vi "Finish.vi"   [LabVIEW 2011]
doc: "This VI is called just before exiting. It is expected to close I/O refnum, save collected data, etc."
types:
  T1 = typedef "WPI_JoystickDevRef.ctl" = cluster{"Device":T2}
  T2 = typedef "WPI_JoystickDeviceEnum.ctl" = enum16{"USB 1", "USB 2", "USB 3", "USB 4", "Kinect 1", "Kinect 2"}
  T3 = typedef "WPI_MotorControlDeviceRef.ctl" = cluster{"DeviceStatus":errorcluster, "Type":enum16{"PWM", "CAN"}, "PWM":cluster{"Digital Module":T4, "PWM Channel":T5, "DeadBand":T6}, "CAN":cluster{"Device Number":u8, "Control Mode":T7, "Semaphore":T8, "Max Vout":dbl}, "Invert":bool, "TransformRef":T9, "InvTransformRef":T9}
  T4 = typedef "FPGA_TypedefDigitalModule.ctl" = enum16{"Digital Module 1", "Digital Module 2"}
  T5 = typedef "FPGA_DIOPWMChannel.ctl" = enum8{"PWM 1", "PWM 2", "PWM 3", "PWM 4", "PWM 5", "PWM 6", "PWM 7", "PWM 8", "PWM 9", "PWM 10", "Invalid"}
  T6 = typedef "WPI_PWMDeadband.ctl" = cluster{"Name":string, "maxPositivePwm":i32, "minPositivePwm":i32, "centerPwm":i32, "maxNegativePwm":i32, "minNegativePwm":i32, "angularRange":u16}
  T7 = typedef "WPI_CANJaguar_ControlMode.ctl" = enum8{"Percent VBus", "Current", "Speed", "Position", "Voltage"}
  T8 = typedef "Semaphore RefNum" = refnum<k1>
  T9 = typedef "WPI_PWMTransform_ConPane.ctl" = refnum<vi>
  T10 = typedef "WPI_AnalogChannelDevRef.ctl" = cluster{"DevStatus":errorcluster, "Analog Module":T11, "Analog Channel":T12}
  T11 = typedef "FPGA_TypedefAnalogModule.ctl" = enum16{"Analog Module 1", "Analog Module 2"}
  T12 = typedef "FPGA_AIChannel.ctl" = enum8{"AI 1", "AI 2", "AI 3", "AI 4", "AI 5", "AI 6", "AI 7", "AI 8", "Invalid"}
  T13 = typedef "WPI_RelayDevRef.ctl" = cluster{"DevStatus":errorcluster, "Relay Channel":T14, "Digital Module":T4, "Relay Direction":T15}
  T14 = typedef "FPGA_DIORelayChannel.ctl" = enum8{"Relay 1", "Relay 2", "Relay 3", "Relay 4", "Relay 5", "Relay 6", "Relay 7", "Relay 8", "Invalid"}
  T15 = typedef "WPI_RelayDirection.ctl" = enum16{"Both directions", "Forward only", "Reverse only"}
  T16 = typedef "WPI_RobotDriveDevRef.ctl" = cluster{"DevStatus":errorcluster, "Motors[]":T3[], "Square Inputs":bool, "Max Output":dbl, "Isochronous":bool}
  T17 = typedef "WPI_CameraDevRef.ctl" = cluster{"Camera Address":string, "CameraStatus":errorcluster, "Acquire Image Notifier":refnum<notifier>}
  T18 = typedef "WPI_ServoDeviceRef.ctl" = cluster{"DeviceStatus":errorcluster, "Digital Module":T4, "PWM Channel":T5, "DeadBand":T6}
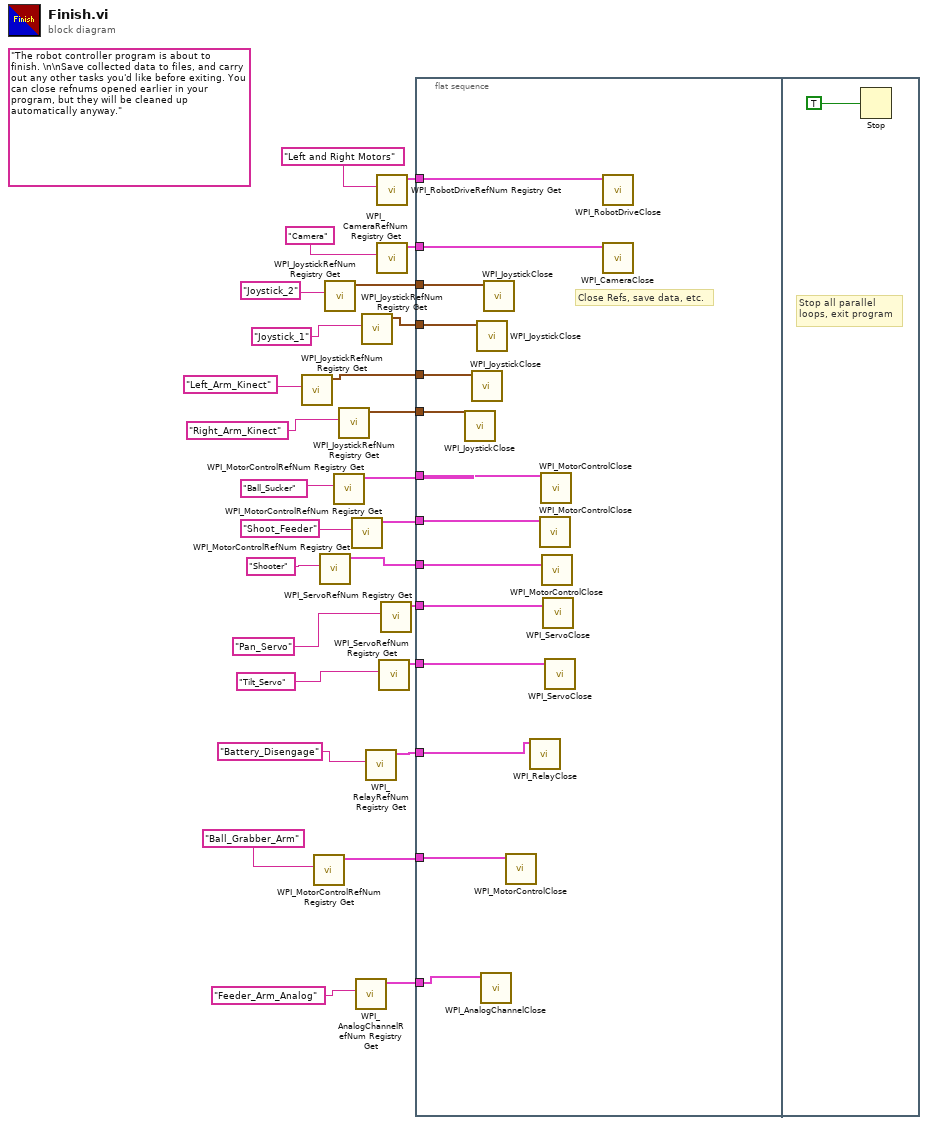
[diagram p0: block diagram]
diagram:
  (unwired) "The robot controller program is about to finish. \n\nSave collected data to files, and carry out any other tasks you'd like before exiting. You can close refnums opened earlier in your program, but they will be cleaned up automatically anyway."
  n1 = call <vilib>:"WPI_JoystickRefNum Registry Get.vi"("refnum name"="Left_Arm_Kinect") -> ("JoystickDevRef"=w6:T1)  [unwired: 1 in, 9 out]
  n2 = call <vilib>:"WPI_MotorControlRefNum Registry Get.vi"("refnum name"="Ball_Grabber_Arm") -> ("MotorControlDevRef"=w3:T3)  [unwired: 9 in, 1 out]
  n3 = call <vilib>:"WPI_MotorControlRefNum Registry Get.vi"("refnum name"="Shooter") -> ("MotorControlDevRef"=w17:T3)  [unwired: 9 in, 1 out]
  n4 = call <vilib>:"WPI_JoystickRefNum Registry Get.vi"("refnum name"="Joystick_2") -> ("JoystickDevRef"=w23:T1)  [unwired: 1 in, 9 out]
  n5 = call <vilib>:"WPI_MotorControlRefNum Registry Get.vi"("refnum name"="Ball_Sucker") -> ("MotorControlDevRef"=w22:T3)  [unwired: 9 in, 1 out]
  n6 = call <vilib>:"WPI_JoystickRefNum Registry Get.vi"("refnum name"="Right_Arm_Kinect") -> ("JoystickDevRef"=w5:T1)  [unwired: 1 in, 9 out]
  n7 = call <vilib>:"WPI_MotorControlRefNum Registry Get.vi"("refnum name"="Shoot_Feeder") -> ("MotorControlDevRef"=w19:T3)  [unwired: 9 in, 1 out]
  n8 = call <vilib>:"WPI_AnalogChannelRefNum Registry Get.vi"("refnum name"="Feeder_Arm_Analog") -> ("AIDeviceRef"=w9:T10)  [unwired: 9 in, 1 out]
  n9 = call <vilib>:"WPI_JoystickRefNum Registry Get.vi"("refnum name"="Joystick_1") -> ("JoystickDevRef"=w11:T1)  [unwired: 1 in, 9 out]
  n10 = call <vilib>:"WPI_RelayRefNum Registry Get.vi"("refnum name"="Battery_Disengage") -> ("RelayDevRef"=w1:T13)  [unwired: 9 in, 1 out]
  n11 = call <vilib>:"WPI_RobotDriveRefNum Registry Get.vi"("refnum name"="Left and Right Motors") -> ("RobotDriveDevRef"=w27:T16)  [unwired: 1 in, 9 out]
  n12 = call <vilib>:"WPI_CameraRefNum Registry Get.vi"("refnum name"="Camera") -> ("CameraDevRef"=w26:T17)  [unwired: 1 in, 9 out]
  n13 = call <vilib>:"WPI_ServoRefNum Registry Get.vi"("refnum name"="Tilt_Servo") -> ("ServoDeviceRef"=w14:T18)  [unwired: 1 in, 9 out]
  n14 = call <vilib>:"WPI_ServoRefNum Registry Get.vi"("refnum name"="Pan_Servo") -> ("ServoDeviceRef"=w15:T18)  [unwired: 1 in, 9 out]
  n15 = flat-sequence {
    tunnel: w27 -> [w42]
    tunnel: w26 -> [w41]
    tunnel: w23 -> [w40]
    tunnel: w22 -> [w39]
    tunnel: w19 -> [w38]
    tunnel: w17 -> [w37]
    tunnel: w15 -> [w36]
    tunnel: w14 -> [w35]
    tunnel: w11 -> [w34]
    tunnel: w9 -> [w33]
    tunnel: w6 -> [w32]
    tunnel: w5 -> [w31]
    tunnel: w3 -> [w30]
    tunnel: w1 -> [w29]
    frame #0 {
      # "Close Refs, save data, etc."
      n16 = call <vilib>:"WPI_JoystickClose.vi"("JoystickDevRef"=w31) -> ()  [unwired: 11 out]
      n17 = call <vilib>:"WPI_JoystickClose.vi"("JoystickDevRef"=w32) -> ()  [unwired: 11 out]
      n18 = call <vilib>:"WPI_JoystickClose.vi"("JoystickDevRef"=w34) -> ()  [unwired: 11 out]
      n19 = call <vilib>:"WPI_AnalogChannelClose.vi"("AIDeviceRef"=w33) -> ()  [unwired: 10 in, 1 out]
      n20 = call <vilib>:"WPI_JoystickClose.vi"("JoystickDevRef"=w40) -> ()  [unwired: 11 out]
      n21 = call <vilib>:"WPI_MotorControlClose.vi"("MotorControlDevRef"=w30) -> ()  [unwired: 10 in, 1 out]
      n22 = call <vilib>:"WPI_RelayClose.vi"("RelayDevRef"=w29) -> ()  [unwired: 10 in, 1 out]
      n23 = call <vilib>:"WPI_MotorControlClose.vi"("MotorControlDevRef"=w38) -> ()  [unwired: 10 in, 1 out]
      n24 = call <vilib>:"WPI_MotorControlClose.vi"("MotorControlDevRef"=w39) -> ()  [unwired: 10 in, 1 out]
      n25 = call <vilib>:"WPI_MotorControlClose.vi"("MotorControlDevRef"=w37) -> ()  [unwired: 10 in, 1 out]
      n26 = call <vilib>:"WPI_ServoClose.vi"("MotorControlDevRef"=w36) -> ()  [unwired: 1 in, 10 out]
      n27 = call <vilib>:"WPI_ServoClose.vi"("MotorControlDevRef"=w35) -> ()  [unwired: 1 in, 10 out]
      n28 = call <vilib>:"WPI_RobotDriveClose.vi"("RobotDriveDevRef"=w42) -> ()  [unwired: 1 in, 10 out]
      n29 = call <vilib>:"WPI_CameraClose.vi"("CameraDevRef"=w41) -> ()  [unwired: 1 in, 10 out]
    }
    frame #1 {
      # "Stop all parallel\nloops, exit program"
      n30 = Stop(stop? (T)=TRUE ("Quit")) -> ()
    }
  }
